vi "expand bool for MUX80 config.vi"(7 "RegEx":string, 8 "Input Config Str":string, 11 "NumChannels":i32) -> (2 "Output Config Arr":bool[](array[boolean]))   [LabVIEW 2020]
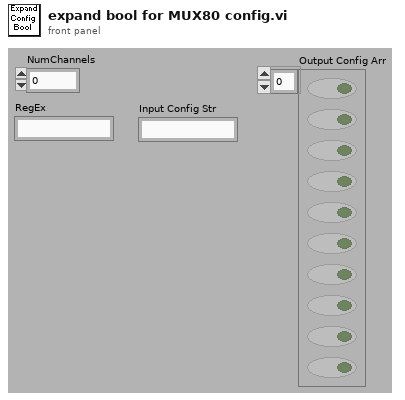
[diagram p1: front panel]
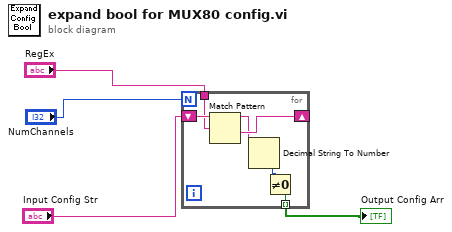
[diagram p0: block diagram]
diagram:
  n1 = for {
    N: "NumChannels" -> [_]
    shift-right: [w8] -> _
    shift-left: "Input Config Str" -> [w10]
    tunnel: "RegEx" -> [w9]
    tunnel: [w5] -> w1 mode=indexing
    n2 = Match Pattern(string=w10, regular expression=w9) -> (before substring=w7:string, after substring=w8:string)  [unwired: 1 in, 2 out]
    n3 = Decimal String To Number(string=w7) -> (number=w6:i32)  [unwired: 2 in, 1 out]
    n4 = Not Equal To 0?(x=w6) -> (x != 0?=w5:bool)
  }
  "Output Config Arr" <- w1
